vi "Get COMM List.vi"(8 "error in (no error)":errorcluster, 11 "CCD in":refnum<class "CCD.lvclass">) -> (0 "error out":errorcluster, 2 "COMM List":string[](array[string]), 3 "CCD out":refnum<class "CCD.lvclass">)   [LabVIEW 2016, in "CCD.lvlib" / "CCD.lvclass"]
uses:
  <userlib>/Common Components/Hardware/CCD/CCD/CCD.lvclass
  <userlib>/Common Components/Hardware/Abstract Hardware/Hardware.lvclass
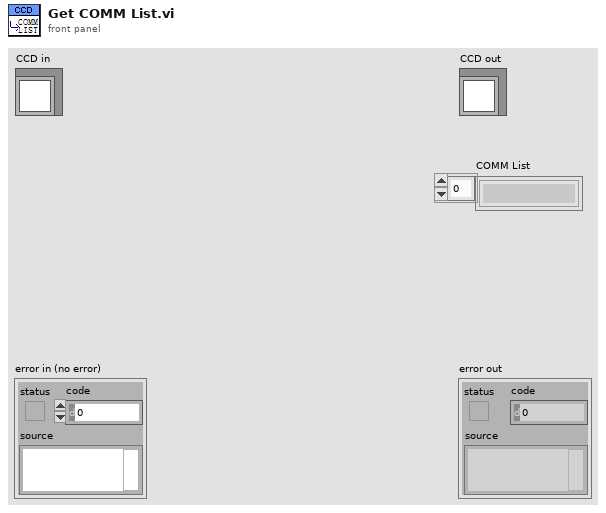
[diagram p1: front panel]
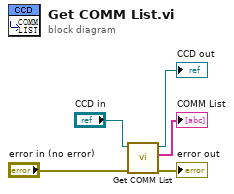
[diagram p0: block diagram]
diagram:
  n1 = call-parent "Get COMM List.vi"("error in (no error)"="error in (no error)", "Hardware in"="CCD in") -> ("error out"=→"error out":errorcluster, "COMM List"=→"COMM List":string[], "Hardware out"=→"CCD out":refnum<class "CCD.lvclass">)  [unwired: 7 in]
